vi "Read Defaults from INI File.vi"(8 "error in (no error)":errorcluster, 11 "Toggle 6 in":refnum<class "Toggle 6.lvclass">) -> (0 "error out":errorcluster, 3 "Toggle 6 out":refnum<class "Toggle 6.lvclass">)   [LabVIEW 2020, in "Toggle 6.lvclass"]
doc: "Reads default values from ini file and put it into the \"registers to write\" array in the device class."
uses:
  Toggle 6.lvclass
  Controls/Register to Write.ctl
  <vilib>/Utility/config.llb/Read Key (U32).vi
  <vilib>/Utility/config.llb/NI_LVConfig.lvlib
  PIC-device/PIC-Device.lvclass
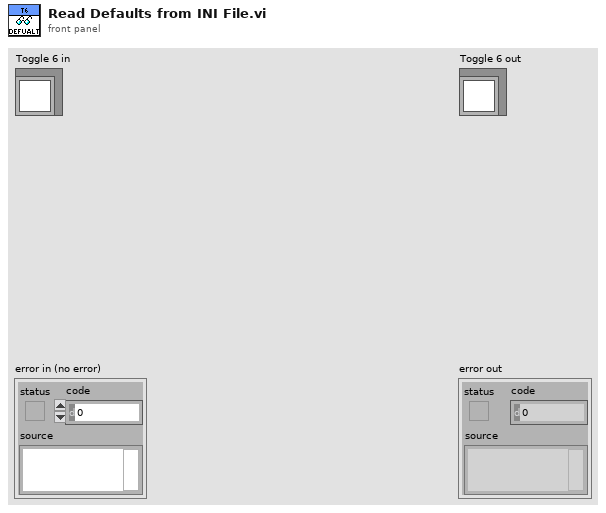
[diagram p1: front panel]
types:
  T1 = typedef "PIC-Device.lvclass/Register to Write.ctl" = cluster{"Register":u32, "Value":u32, "Dev Address":u32, "Physical Adress":u32}
  T2 = typedef "NI_LVConfig.lvlib/Config Data RefNum.ctl" = refnum<k1>
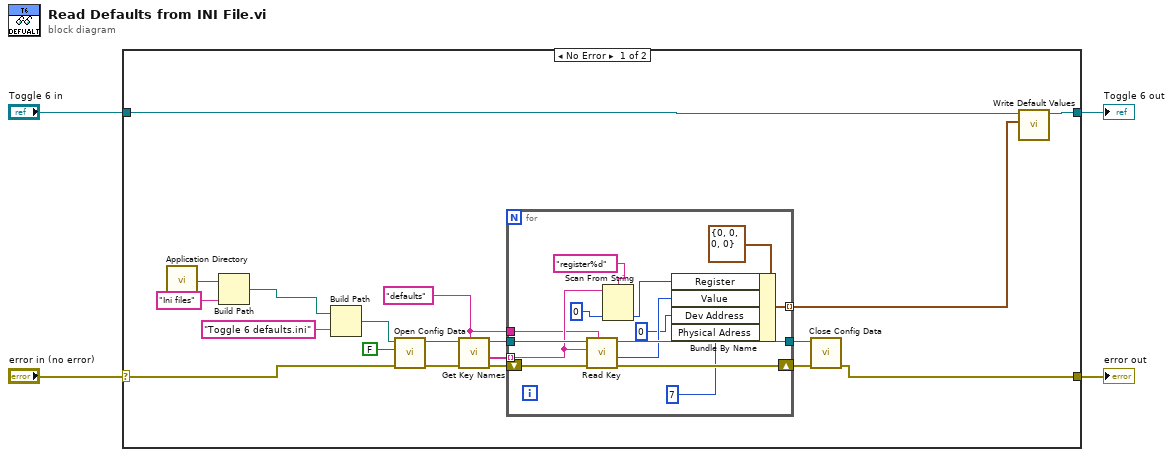
[diagram p0: block diagram]
diagram:
  n1 = case shown="No Error" "error in (no error)" {
    selector: "error in (no error)" -> [w23 w39]
    tunnel: [w9 w39] -> w3
    tunnel: [w7 w38] -> w1
    tunnel: "Toggle 6 in" -> [w6 w38]
    frame No Error {
      w12 = "defaults" ("section")
      n2 = call <vilib>:"Application Directory.vi"() -> ("Application Directory"=w22:path)
      n3 = Build Path(base path=w22, name or relative path="Ini files") -> (appended path=w5:path)
      n4 = Build Path(base path=w5, name or relative path="Toggle 6 defaults.ini") -> (appended path=w19:path)
      n5 = call <vilib>:"Open Config Data.vi"("error in (no error)"=w23, "create file if necessary (T)"=FALSE, "configuration file path"=w19) -> ("error out"=w17:errorcluster, "refnum"=w16:T2)  [unwired: 6 in, 1 out]
      n6 = call <vilib>:"Get Key Names.vi"("section"=w12, "error in (no error)"=w17, "refnum"=w16) -> ("error out"=w15:errorcluster, "key names"=w13:string[], "refnum out"=w14:T2)  [unwired: 5 in, 1 out]
      n7 = for {
        tunnel: w14 -> [w36]
        tunnel: w13 -> [w34] mode=indexing
        tunnel: w12 -> [w33]
        shift-right: [w32] -> w11
        shift-left: w15 -> [w35]
        tunnel: [w31] -> w10
        tunnel: [w28] -> w8 mode=indexing
        n8 = call-poly <vilib>:"Read Key.vi"("section"=w33, "error in (no error)"=w35, "key"=w34, "refnum"=w36) -> ("error out"=w32:errorcluster, "value"=w29:u32, "refnum out"=w31:T2)  [unwired: 4 in, 1 out]
        n9 = Scan From String(format string="register%d", input string=w34, default 1=u32 0) -> (output 1=w30:u32)  [unwired: 2 in, 3 out]
        n10 = Bundle By Name(cluster=T1 {"Register"=0, "Value"=0, "Dev Address"=0, "Physical Adress"=0} ("Cluster"), "Register"=w30, "Value"=w29, "Dev Address"=u32 0 ("Adress"), "Physical Adress"=u32 7) -> (w28:T1)
      }
      n11 = call <vilib>:"Close Config Data.vi"("error in (no error)"=w11, "refnum"=w10) -> ("error out"=w9:errorcluster)  [unwired: 8 in, 1 out]
      n12 = call-dynamic "Write Default Values.vi"("Default Values"=w8, "Toggle 6 in"=w6) -> ("Toggle 6 out"=w7:refnum<class "Toggle 6.lvclass">)  [unwired: 9 in]
    }
    frame Error {
    }
  }
  "error out" <- w3
  "Toggle 6 out" <- w1
